vi "Destroy.vi"(8 "error in (no error)":errorcluster, 11 "file handler in":refnum<class "File Handler.lvclass">) -> (0 "error out":errorcluster)   [LabVIEW 2018, in "Logging.lvlib" / "File Handler.lvclass"]
uses:
  File Handler.lvclass
  File Handler.lvclass/File Handler.ctl
panel:
  # "Connector Pane"
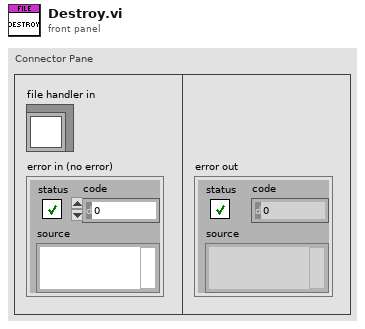
[diagram p1: front panel]
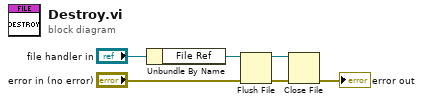
[diagram p0: block diagram]
diagram:
  n1 = Unbundle By Name("file handler in") -> ("File Ref"=w2:refnum<file>)
  n2 = Flush File(refnum=w2, error in="error in (no error)") -> (refnum out=w1:refnum<file>, error out=w3:errorcluster)
  n3 = Close File(refnum=w1, error in=w3) -> (error out=→"error out":errorcluster)  [unwired: 1 out]
